vi "Vision Test.vi"(11 "CameraDevRef":T2) -> (2 "Camera Image":T1(plugin-control), 3 "Particle Measurements (Pixels)":dbl[][](array[numeric]) format="%.2f")   [LabVIEW 2013]
uses:
  <vilib>/Rock Robotics/WPI/Camera/WPI_CameraDevRef.ctl
panel:
  in  "error in (no error)":errorcluster
  out "4":bool
  out "3":bool
  out "1":bool
  out "2":bool
  out "x-y":dbl
  out "error out":errorcluster
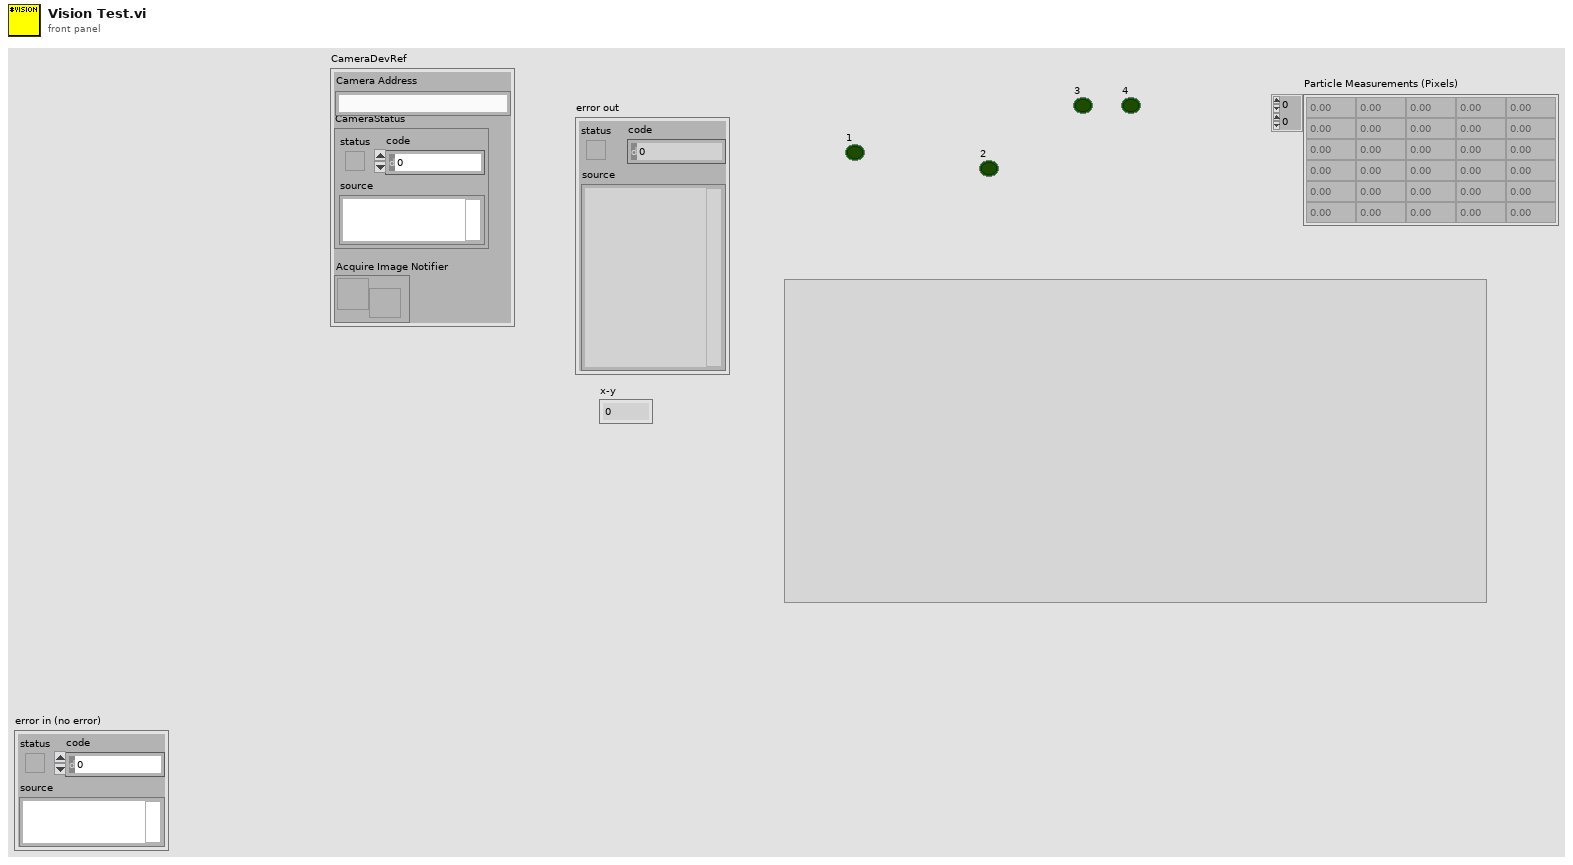
[diagram p1: front panel]
types:
  T1 = typedef "IMAQ Image.ctl" = refnum<image>
  T2 = typedef "WPI_CameraDevRef.ctl" = cluster{"Camera Address":string, "CameraStatus":errorcluster, "Acquire Image Notifier":refnum<notifier>}
  T3 = typedef "Image Type" = u32
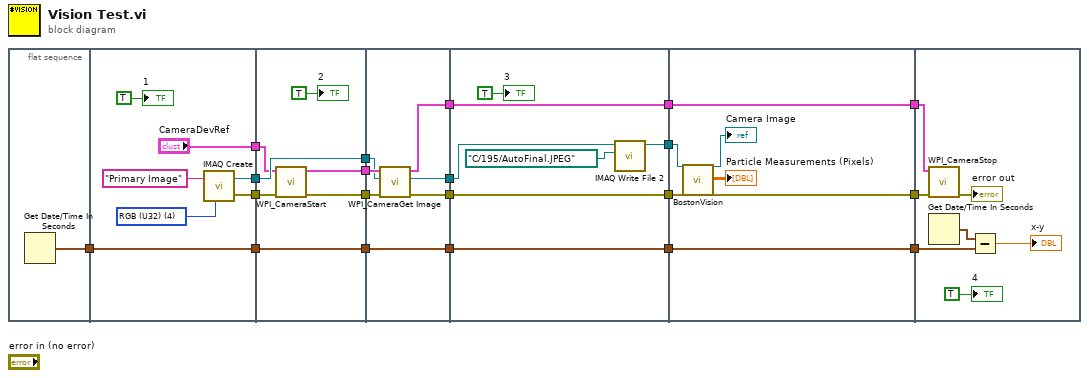
[diagram p0: block diagram]
diagram:
  n1 = flat-sequence {
    tunnel: [w21] -> w20
    tunnel: [w26] -> w18
    tunnel: w20 -> [w26]
    tunnel: [w25] -> w16
    tunnel: ["CameraDevRef"] -> w15
    tunnel: [w22] -> w13
    tunnel: w18 -> [w35]
    tunnel: [w35] -> w17
    tunnel: w16 -> [w30]
    tunnel: w15 -> [w29]
    tunnel: [w32] -> w14
    tunnel: w13 -> [w34]
    tunnel: [w34] -> w12
    tunnel: [w31] -> w6
    tunnel: w17 -> [w42]
    tunnel: [w42] -> w11
    tunnel: [w41] -> w9
    tunnel: w14 -> [w39]
    tunnel: w12 -> [w38]
    tunnel: [w37] -> w8
    tunnel: w6 -> [w40]
    tunnel: [w36] -> w3
    tunnel: w11 -> [w49]
    tunnel: [w49] -> w10
    tunnel: w9 -> [w44]
    tunnel: w8 -> [w47]
    tunnel: [w47] -> w7
    tunnel: [w46] -> w4
    tunnel: w3 -> [w46]
    tunnel: [w43] -> w2
    tunnel: w10 -> [w56]
    tunnel: [w56] -> w19
    tunnel: w7 -> [w53]
    tunnel: [w55] -> w5
    tunnel: w4 -> [w55]
    tunnel: w2 -> [w54]
    tunnel: [w50] -> w1
    tunnel: w19 -> [w61]
    tunnel: w5 -> [w58]
    tunnel: w1 -> [w59]
    frame #0 {
      n2 = Get Date/Time In Seconds() -> (seconds since 1Jan1904=w21:timestamp)
    }
    frame #1 {
      w27 = T3 4 items=["Grayscale (U8)", "Grayscale (I16)", "Grayscale (SGL)", "Complex (CSG)", "RGB (U32)", "HSL (U32)", "RGB (U64)"] ("Image Type")
      n3 = call "IMAQ Create"("Image Name"="Primary Image", "Image Type"=w27) -> ("New Image"=w22:T1, "error out"=w25:errorcluster)  [unwired: 2 in, 1 out]
      "1" <- TRUE
    }
    frame #2 {
      n4 = call <vilib>:"WPI_CameraStart.vi"("error in (no error)"=w30, "CameraDevRef"=w29) -> ("error out"=w31:errorcluster, "CameraDevRef Out"=w32:T2)  [unwired: 8 in]
      "2" <- TRUE
    }
    frame #3 {
      n5 = call <vilib>:"WPI_CameraGet Image.vi"("error in (no error)"=w40, "Image"=w38, "CameraDevRef"=w39) -> ("error out"=w37:errorcluster, "Image Out"=w41:T1, "CameraDevRef Out"=w36:T2)  [unwired: 6 out]
    }
    frame #4 {
      n6 = call-poly "IMAQ Write File 2"("File Path"=path "C:/195/AutoFinal.JPEG", "Image"=w44) -> ("Image Out (duplicate)"=w43:T1)  [unwired: 8 in, 1 out]
      "3" <- TRUE
    }
    frame #5 {
      n7 = call "BostonVision.vi"("Image In"=w54, "error in"=w53) -> ("Image Out"=→"Camera Image":T1, "Particle Measurements (Pixels)"=→"Particle Measurements (Pixels)":dbl[][], "error out"=w50:errorcluster)  [unwired: 23 in]
    }
    frame #6 {
      n8 = call <vilib>:"WPI_CameraStop.vi"("error in (no error)"=w59, "CameraDevRef"=w58) -> ("error out"=→"error out":errorcluster)  [unwired: 8 in, 1 out]
      n9 = Get Date/Time In Seconds() -> (seconds since 1Jan1904=w63:timestamp)
      n10 = Subtract(x=w63, y=w61) -> (x-y=→"x-y":dbl)
      "4" <- TRUE
    }
  }
